vi "load binary file.vi"() -> ()   [LabVIEW 2013, in "Binary datalogger runtime.lvclass"]
uses:
  Binary datalogger runtime.lvclass
  data cache.ctl
  <vilib>/NI/Tag Bus/table/data table.ctl
  <vilib>/NI/Tag Bus/dictionary/full data dictionary.ctl
  <vilib>/NI/Tag Bus/table/data table.lvlib
  <vilib>/NI/Tag Bus/dictionary/data dictionary.lvclass
panel:
  in  "path":path
  out "error out":errorcluster
  out "version":string
  out "remaining string":string
  out "dictionary":T1
  out "data":T2[](array[typedef])
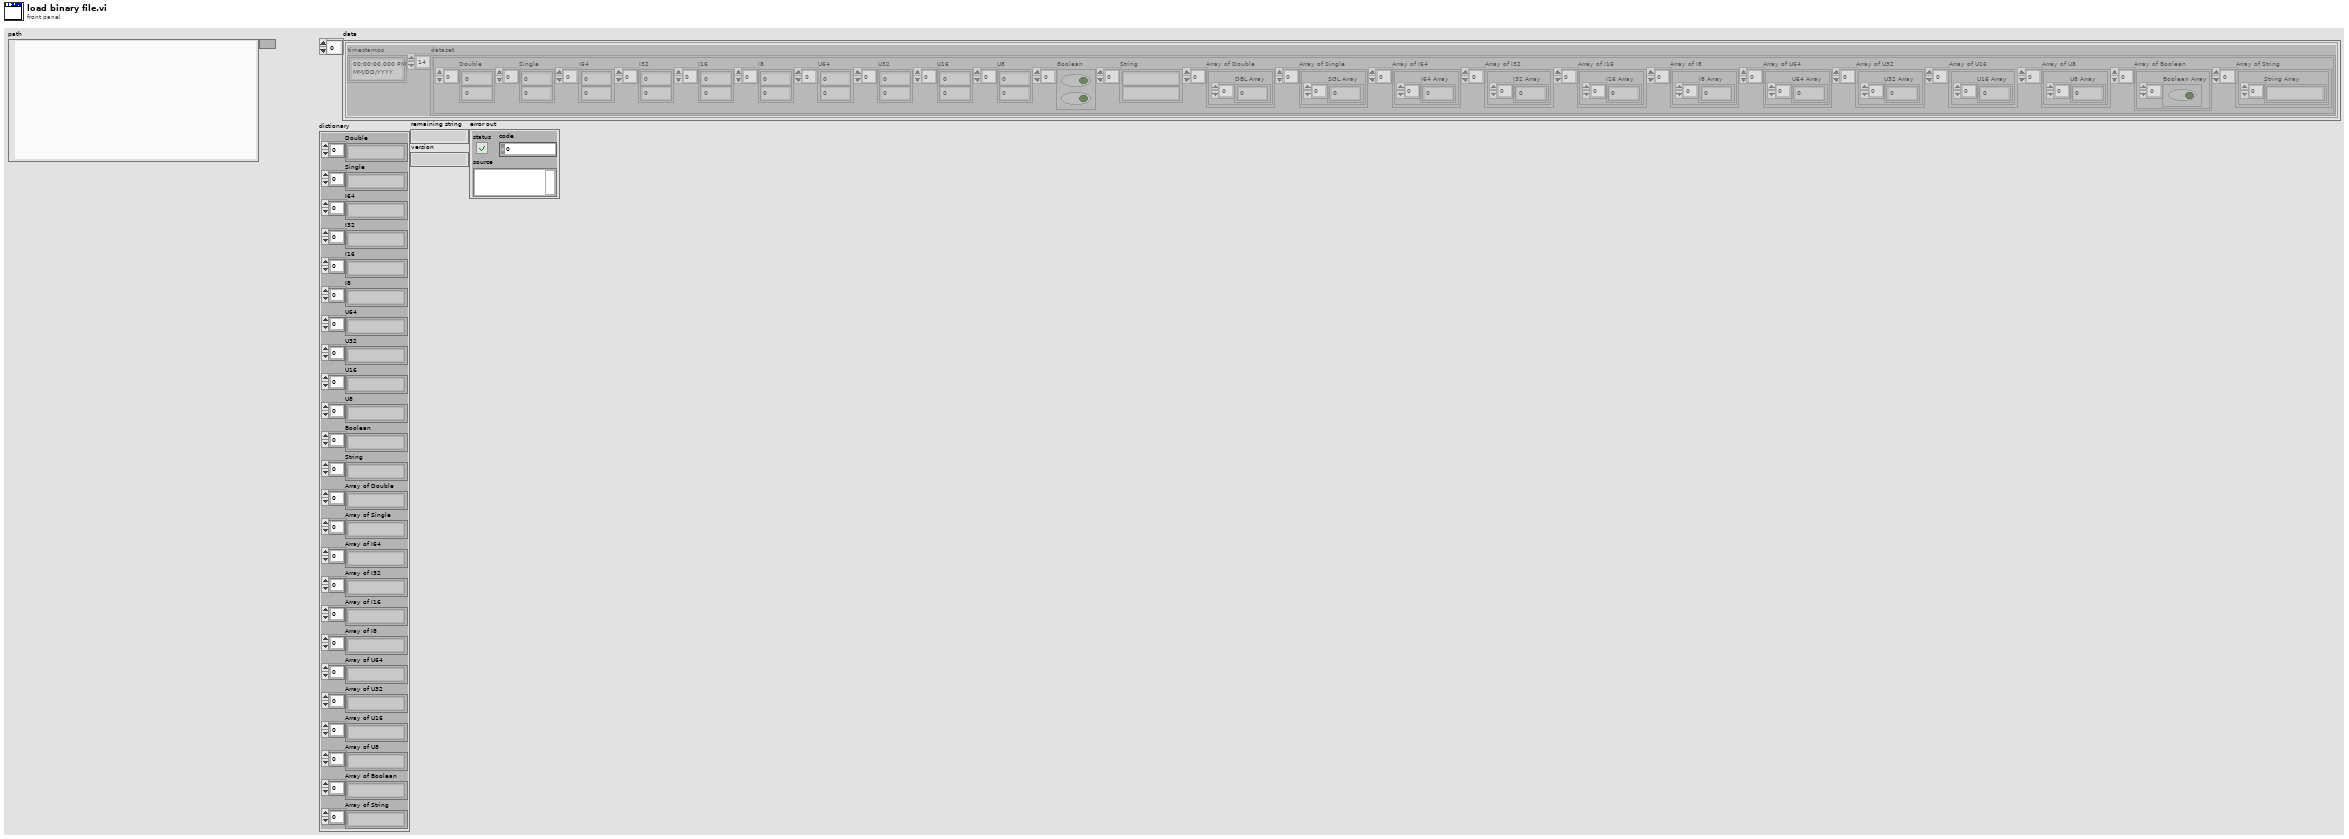
[diagram p1: front panel]
types:
  T1 = typedef "tag bus.lvlib/data dictionary.lvclass/full data dictionary.ctl" = cluster{"Double":string[], "Single":string[], "I64":string[], "I32":string[], "I16":string[], "I8":string[], "U64":string[], "U32":string[], "U16":string[], "U8":string[], "Boolean":string[], "String":string[], "Array of Double":string[], "Array of Single":string[], "Array of I64":string[], "Array of I32":string[], "Array of I16":string[], "Array of I8":string[], "Array of U64":string[], "Array of U32":string[], "Array of U16":string[], "Array of U8":string[], "Array of Boolean":string[], "Array of String":string[]}
  T2 = typedef "Binary datalogger runtime.lvclass/data cache.ctl" = cluster{"timestamps":timestamp[], "dataset":T3[]}
  T3 = typedef "tag bus.lvlib/data table.lvlib/data table.ctl" = cluster{"Double":dbl[], "Single":sgl[], "I64":i64[], "I32":i32[], "I16":i16[], "I8":i8[], "U64":u64[], "U32":u32[], "U16":u16[], "U8":u8[], "Boolean":bool[], "String":string[], "Array of Double":cluster{"DBL Array":dbl[]}[], "Array of Single":cluster{"SGL Array":sgl[]}[], "Array of I64":cluster{"I64 Array":i64[]}[], "Array of I32":cluster{"I32 Array":i32[]}[], "Array of I16":cluster{"I16 Array":i16[]}[], "Array of I8":cluster{"I8 Array":i8[]}[], "Array of U64":cluster{"U64 Array":u64[]}[], "Array of U32":cluster{"U32 Array":u32[]}[], "Array of U16":cluster{"U16 Array":u16[]}[], "Array of U8":cluster{"U8 Array":u8[]}[], "Array of Boolean":cluster{"Boolean Array":bool[]}[], "Array of String":cluster{"String Array":string[]}[]}
  T4 = enum16{"open", "replace", "create", "open or create", "replace or create", "replace or create with confirmation"}
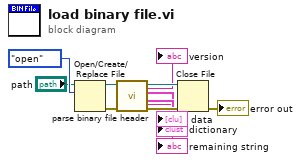
[diagram p0: block diagram]
diagram:
  n1 = Open/Create/Replace File(file path (use dialog)="path", operation (0:open)=T4."open") -> (refnum out=w10:refnum<file>, error out=w7:errorcluster)  [unwired: 4 in, 1 out]
  n2 = call "parse binary file header.vi"("error in"=w7, "Byte Stream File in"=w10) -> ("error out"=w8:errorcluster, "data"=→"data":T2[], "dictionary"=→"dictionary":T1, "Byte Stream File out"=w9:refnum<file>, "remaining string"=→"remaining string":string, "version"=→"version":string)  [unwired: 4 in]
  n3 = Close File(refnum=w9, error in=w8) -> (error out=→"error out":errorcluster)  [unwired: 1 out]
